vi "XML Build Poll Request(N).vi"(2 "XML-Message alt":string, 3 "EVID-Nummern":i32[](array[numeric])) -> (0 "Attribut Name (N)":string[](array[string]), 7 "XML-Message neu":string)   [LabVIEW 2020, in "FT-IR.lvlib" / "TOOLweb Interface.lvlib" / "TOOLweb Interface Hilfs-VIs.lvlib"]
doc: "Fügt an die bisher aufgebauten XML-Poll-Request-Zeilen \"XML-Message alt\" eine Poll-Request-Zeile hinzu, die alle Variablen mit den IDs im Array \"EVID-Nummern\" anfordert.\n\nDer Ausgang \"Attribut Name (N)\" wird zu einem auf gleicher Höhe liegendem XML-Parser verbunden, der damit keine weiteren Informationen benötigt.\n\nDer Ausgangs-String \"XML-Message neu\" wird an ein weiteres XML-Build-VI oder an das abschließende \"XML Build Poll Request Frame\" übergeben, das allen Zeilen gemeinsam mit dem Start-Tag <PollRequest> und dem End-Tag </PollRequest> den Rahmen für eine einzige und damit schnelle XML-Anfrage gibt."
uses:
  TOOLweb Interface Hilfs-VIs.lvlib
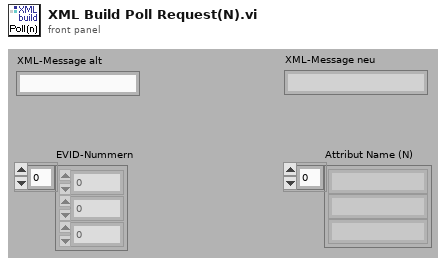
[diagram p1: front panel]
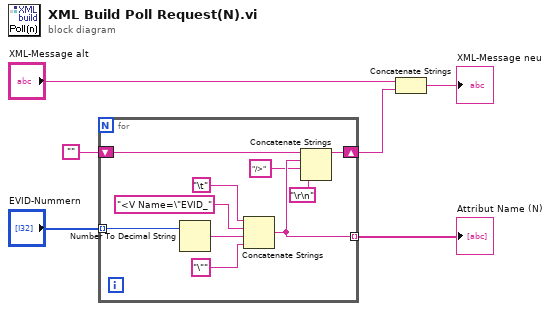
[diagram p0: block diagram]
diagram:
  n1 = for {
    tunnel: "EVID-Nummern" -> [w13] mode=indexing
    shift-right: [w11] -> w1
    shift-left: "" -> [w12]
    tunnel: [w10] -> w2 mode=indexing
    n2 = Number To Decimal String(number=w13) -> (decimal integer string=w15:string)  [unwired: 1 out]
    n3 = Concatenate Strings("\t", "<V Name=\"EVID_" ("Daten (Eingang)"), w15, "\"" ("Daten (Eingang)")) -> (w10:string)
    n4 = Concatenate Strings(w12, w10, "/>" ("Daten (Eingang)"), "\r\n") -> (w11:string)
  }
  "Attribut Name (N)" <- w2
  n5 = Concatenate Strings("XML-Message alt", w1) -> (→"XML-Message neu":string)
